vi "Test Set Row Values.vi"(11 "Test Case In":refnum<class "Test Open Xml.lvclass">) -> (0 "error out":errorcluster, 3 "Test Case Out":refnum<class "Test Open Xml.lvclass">)   [LabVIEW 2025, in "Test Open Xml.lvclass"]
uses:
  Test Open Xml.lvclass
  C:/Program Files/National Instruments/LabVIEW 2025/vi.lib/Astemes/LUnit/Test Case.lvclass
  Source/Cell DataType.ctl
  <vilib>/Astemes/LUnit/Test Case.lvclass/Test Case.ctl
  a710e01d-083e-4ad4-93ae-fbf4f3e7ce4d.vi
  e5169541-515f-4f16-96fe-0f2d3de234a9.vi
  <vilib>/Astemes/LUnit/Append Fail Result.vi
  <vilib>/Astemes/LUnit/Append Pass Result.vi
  <vilib>/Astemes/LUnit/Run In UI.vi
  <vilib>/Utility/error.llb/Clear Errors.vi
  <vilib>/Astemes/LUnit/Test Case.lvclass
  Source/Open Xml.lvlib
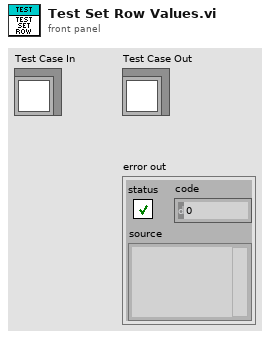
[diagram p1: front panel]
types:
  T1 = typedef "Open Xml.lvlib/Cell DataType.ctl" = enum16{"Void", "Boolean", "Number", "Error", "SharedString", "String", "InlineString", "Date"}
  T2 = cluster{"Number":dbl, "String":string, "Boolean":bool, "Time Stamp":timestamp, "Error":errorcluster}[]
  T3 = cluster{"Number":dbl, "String":string, "Boolean":bool, "Time Stamp":timestamp, "Error":errorcluster}
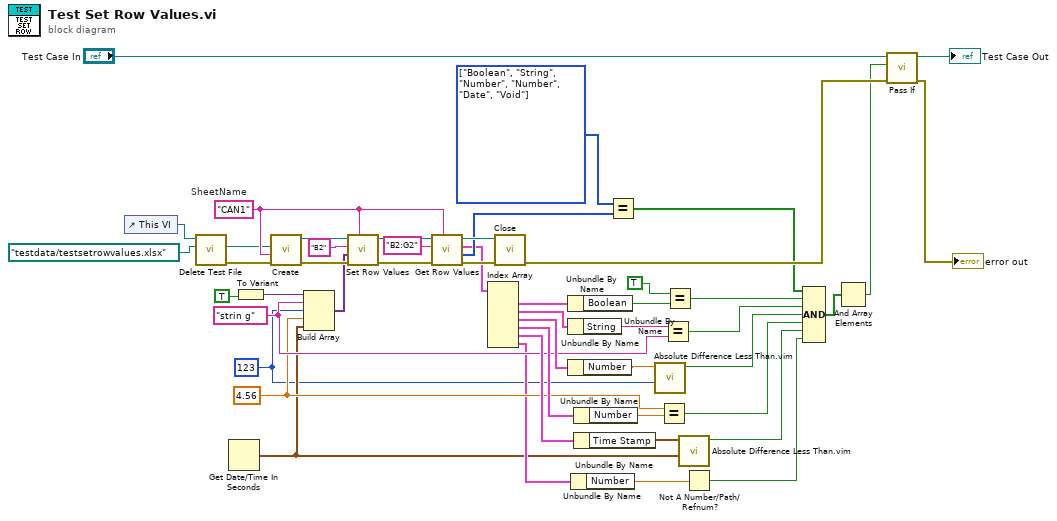
[diagram p0: block diagram]
diagram:
  w30 = T1[] [enum."Boolean", enum."String", enum."Number", enum."Number", enum."Date", enum."Void"] items=["Void", "Boolean", "Number", "Error", "SharedString", "String", "InlineString", "Date"] ("x")
  w13 = 4.56
  w1 = 123
  w15 = "strin g"
  w41 = "CAN1"  # SheetName
  n1 = control-ref of="This VI"() -> (w6:refnum<vi>)
  n2 = call "Delete Test File.vi"("name or relative path"=path "testdata/testsetrowvalues.xlsx", "VI in"=w6) -> ("error out"=w7:errorcluster, "deleted path"=w4:path)  [unwired: 8 in]
  n3 = Get Date/Time In Seconds() -> (seconds since 1Jan1904=w2:timestamp)
  n4 = To Variant(anything=TRUE) -> (Variant=w34:variant)
  n5 = call "Create.vi"("error in"=w7, "SheetName"=w41, "Path"=w4) -> ("error out"=w45:errorcluster, "SpreadsheetDoc"=w46:refnum<k24>)  [unwired: 7 in]
  n6 = Build Array(w34, w15, w1, w13, w2) -> (w22:variant[])
  n7 = call "Set Row Values.vi"("Sheet Name"=w41, "error in"=w45, "Values"=w22, "Cell Address"="B2", "SpreadsheetDoc"=w46) -> ("error out"=w39:errorcluster, "SpreadsheetDoc out"=w38:refnum<k24>)  [unwired: 5 in]
  n8 = call "Get Row Values.vi"("Sheet Name"=w41, "error in"=w39, "Cell Addresses"="B2:G2" ("Cell Address"), "SpreadsheetDoc in"=w38) -> ("error out"=w43:errorcluster, "Types"=w37:T1[], "Cell Values"=w31:T2, "SpreadsheetDoc out"=w42:refnum<k24>)  [unwired: 4 in]
  n9 = Index Array(array=w31) -> (element #1=w29:T3, element #2=w28:T3, element #3=w27:T3, element #4=w26:T3, element #5=w25:T3, element #6=w10:T3)  [unwired: 6 in]
  n10 = call "Close.vi"("error in"=w43, "SpreadsheetDoc"=w42) -> ("error out"=w44:errorcluster)  [unwired: 9 in]
  n11 = Unbundle By Name(w29) -> ("Boolean"=w20:bool)
  n12 = Unbundle By Name(w28) -> ("String"=w17:string)
  n13 = Unbundle By Name(w27) -> ("Number"=w23:dbl)
  n14 = Unbundle By Name(w10) -> ("Number"=w8:dbl)
  n15 = Unbundle By Name(w26) -> ("Number"=w14:dbl)
  n16 = Unbundle By Name(w25) -> ("Time Stamp"=w21:timestamp)
  n17 = Equal?(x=w30, y=w37) -> (x = y?=w36:bool[])
  n18 = call "Absolute Difference Less Than.vim"("Number 2"=w1, "Number 1"=w23) -> ("In Limit"=w3:bool)  [unwired: 9 in]
  n19 = Equal?(x=w13, y=w14) -> (x = y?=w12:bool)
  n20 = Equal?(x=w17, y=w15) -> (x = y?=w16:bool)
  n21 = Equal?(x=TRUE, y=w20) -> (x = y?=w18:bool)
  n22 = call "Absolute Difference Less Than.vim"("Number 2"=w2, "Number 1"=w21) -> ("In Limit"=w11:bool)  [unwired: 9 in]
  n23 = Not A Number/Path/Refnum?(number/path/refnum=w8) -> (NaN/Path/Refnum?=w9:bool)
  n24 = Compound Arithmetic op=AND(w36, w18, w16, w3, w12, w11, w9) -> (w24:bool[])
  n25 = And Array Elements(Boolean array=w24) -> (logical AND=w40:bool)
  n26 = call <vilib>:"Pass If.vi"("error in (no error)"=w44, "Pass?"=w40, "LUnit Test Case In"="Test Case In") -> ("error out"=→"error out":errorcluster, "LUnit Test Case Out"=→"Test Case Out":refnum<class "Test Open Xml.lvclass">)  [unwired: 7 in]
